vi "read_n_samples.vi"(8 "error in (no error)":errorcluster, 11 "Mixture in":refnum<class "Mixture.lvclass">) -> (0 "error out":errorcluster, 2 "n_samples":dbl=1.0, 3 "Mixture out":refnum<class "Mixture.lvclass">)   [LabVIEW 2020, in "Mixture.lvclass"]
uses:
  Mixture.lvclass
  Mixture.lvclass/Mixture.ctl
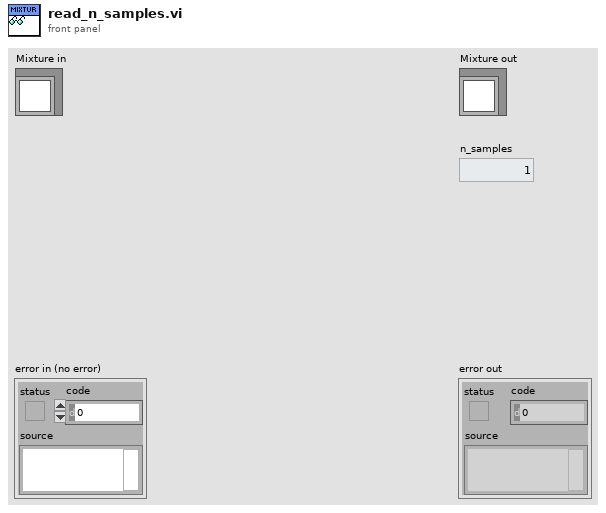
[diagram p1: front panel]
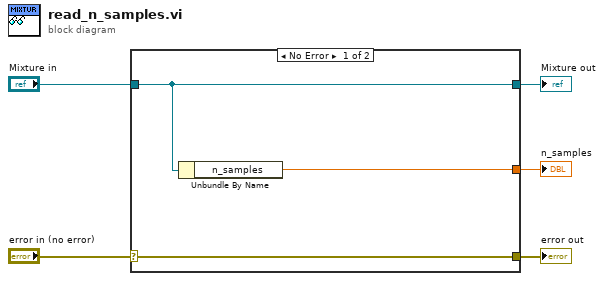
[diagram p0: block diagram]
diagram:
  n1 = case shown="No Error" "error in (no error)" {
    selector: "error in (no error)" -> [w8 w9]
    tunnel: [w8 w9] -> w4
    tunnel: [w7 w10] -> w2
    tunnel: "Mixture in" -> [w7 w10]
    tunnel: [w6 _] -> w1
    frame No Error {
      n2 = Unbundle By Name(w7) -> ("n_samples"=w6:dbl)
    }
    frame Error {
    }
  }
  "error out" <- w4
  "Mixture out" <- w2
  "n_samples" <- w1
